vi "Instrument Manager Loop.vi"(8 "System Control":refnum<queue>, 11 "Instrument Manager":refnum<queue>) -> (0 "error out":errorcluster)   [LabVIEW 2020, in "Rename to match project.lvlib" / "Instrument Manager.lvlib"]
uses:
  Instrument Manager/Instrument Manager.lvlib
  support/Message Queue/Message Cluster.ctl
  Instrument Manager/Instrument State.ctl
  <vilib>/Utility/error.llb/Error Cluster From Error Code.vi
  <vilib>/ErrorRing/Error Ring.xnode
  support/Message Queue/Message Queue.lvlib
  Rename to match project.lvlib
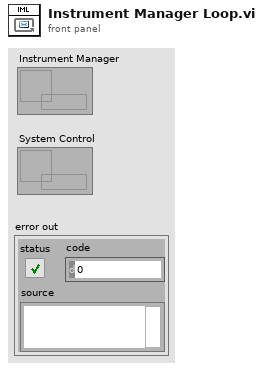
[diagram p1: front panel]
types:
  T1 = typedef "Rename to match project.lvlib/Instrument Manager.lvlib/Instrument State.ctl" = cluster{"VISA Resource":refnum<visa-resource-name>, "Setpoint":dbl, "Running":bool, "Running Since":timestamp, "Example Value Data Point":cluster{"Time Stamp":timestamp, "Value":dbl}, "Sampling Rate (sec/sample)":dbl}
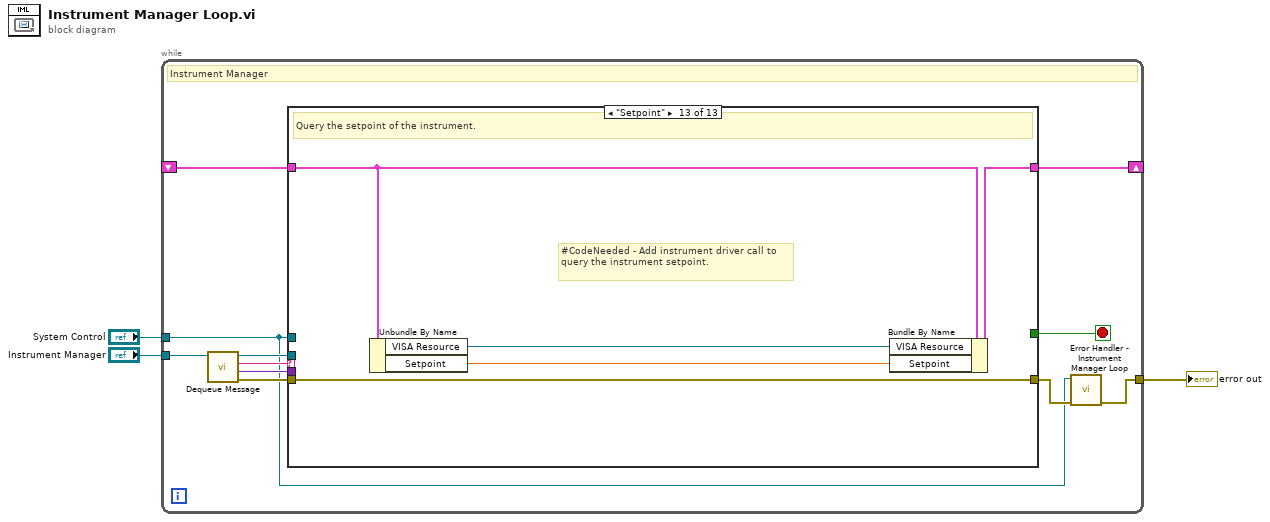
[diagram p0: block diagram]
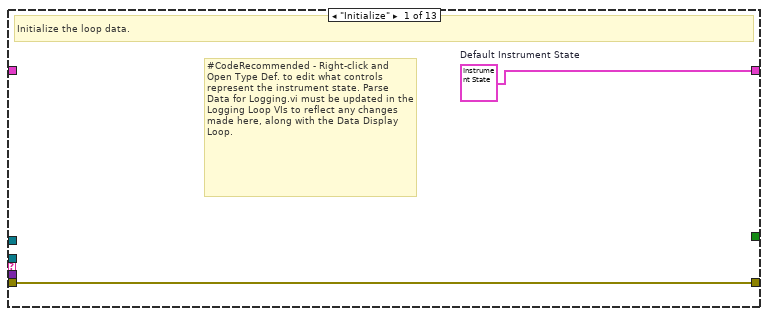
[diagram p2: hidden frame]
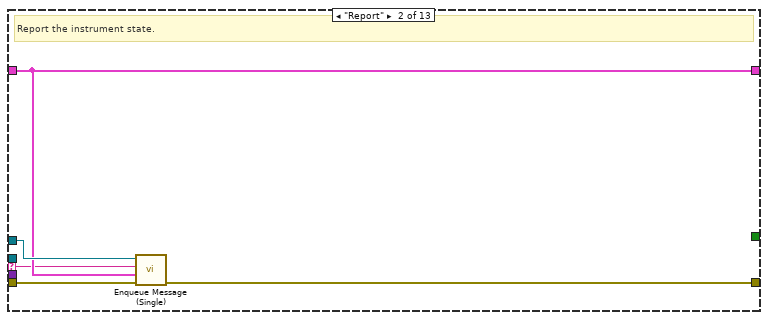
[diagram p3: hidden frame]
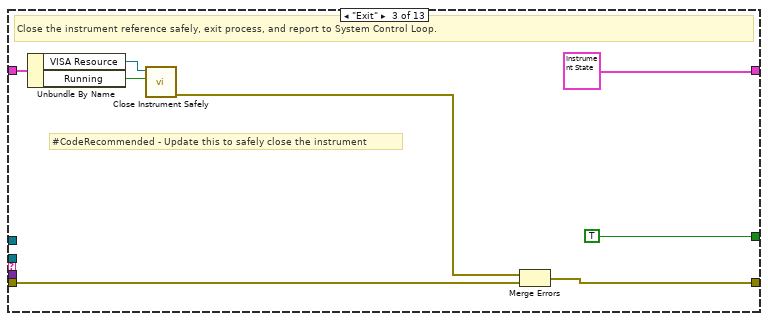
[diagram p4: hidden frame]
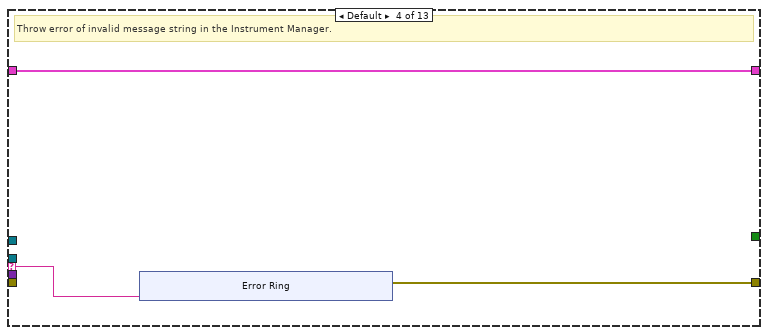
[diagram p5: hidden frame]
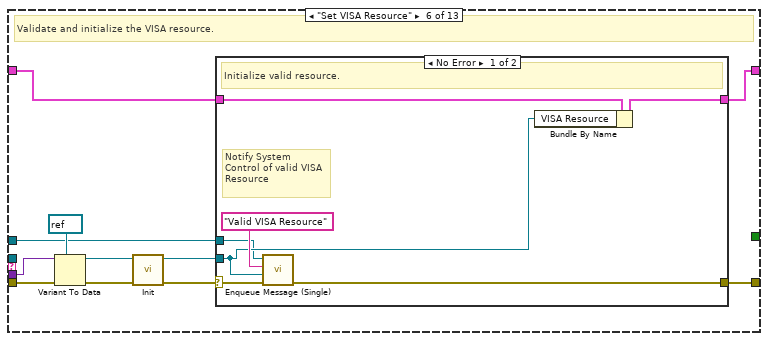
[diagram p7: hidden frame]
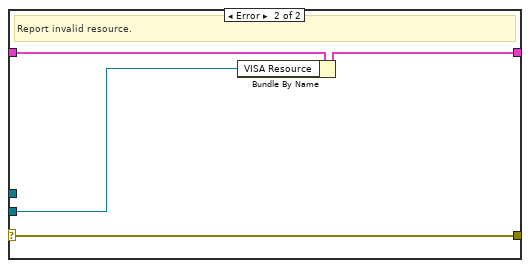
[diagram p8: hidden frame]
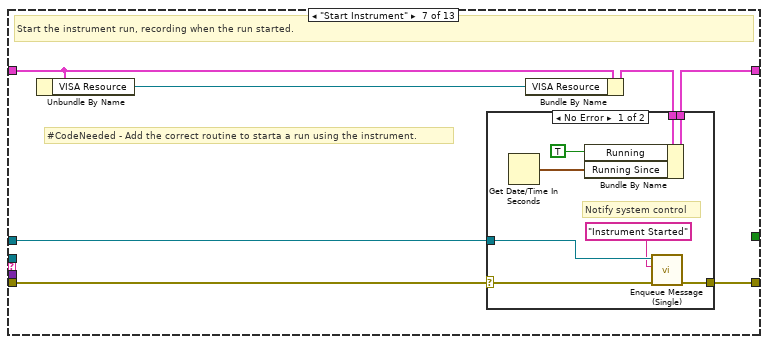
[diagram p9: hidden frame]
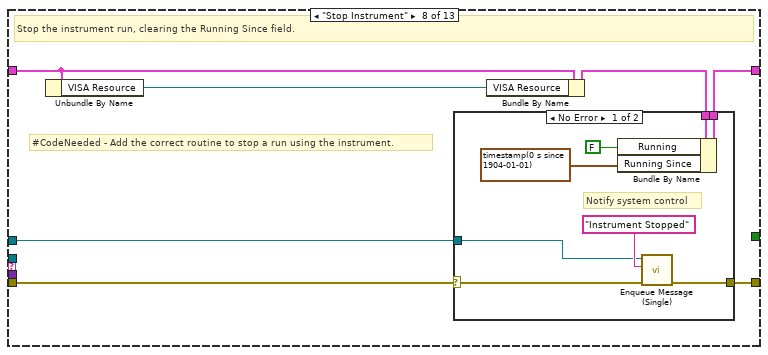
[diagram p11: hidden frame]
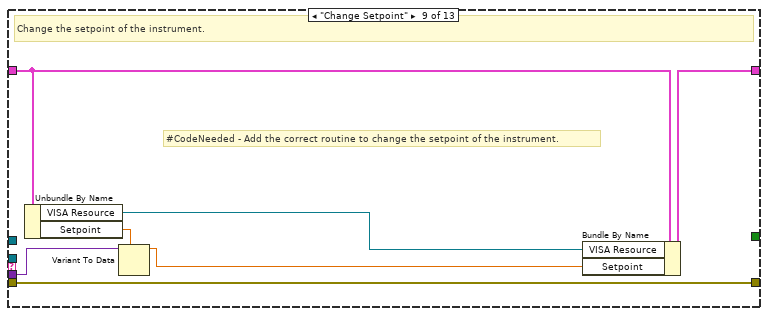
[diagram p13: hidden frame]
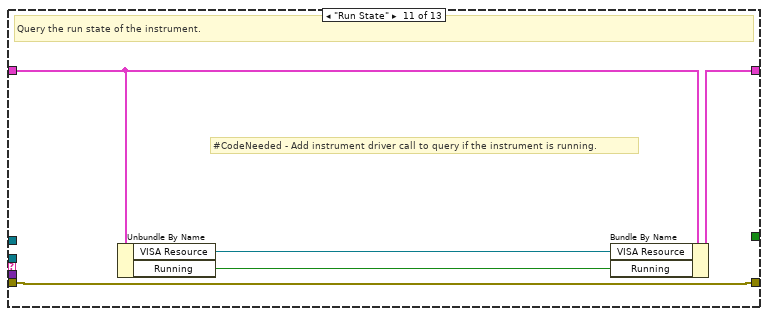
[diagram p15: hidden frame]
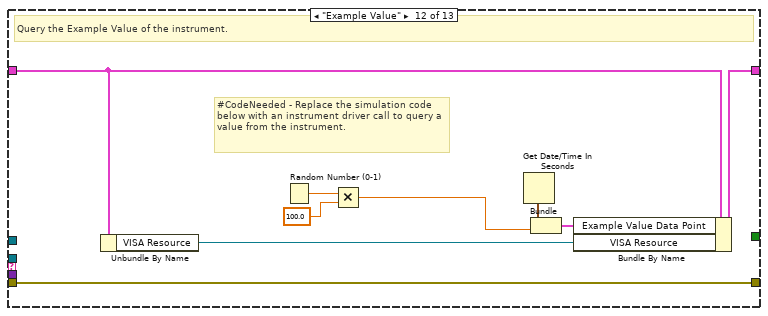
[diagram p16: hidden frame]
diagram:
  n1 = while {
    tunnel: "Instrument Manager" -> [w14]
    tunnel: "System Control" -> [w4]
    tunnel: [w8] -> w1
    shift-right: [w6] -> _
    shift-left: _ -> [w7]
    stop <- w5 stop-if-true
    # "Instrument Manager"
    n2 = call "Dequeue Message.vi"("Message Queue"=w14) -> ("error out"=w10:errorcluster, "Message Data"=w11:variant, "Message"=w13:string, "dup Message Queue"=w12:refnum<queue>)  [unwired: 7 in]
    n3 = case shown="\"Setpoint\"" w13 {
      selector: w13 -> [_ w17 _ w31 _ _ _ _ _ _ _ _ _]
      tunnel: w12 -> [_ _ _ _ _ _ _ _ _ _ _ _ _]
      tunnel: w4 -> [_ w20 _ _ _ w42 w69 w86 _ _ _ _ _]
      tunnel: w11 -> [_ _ _ _ _ w49 _ _ w103 _ _ _ _]
      tunnel: w10 -> [w16 w21 w24 _ w40 w48 w67 w84 w99 w106 w110 w116 w125]
      tunnel: [w16 w19 w23 w30 w40 w52 w70 w87 w99 w106 w110 w116 w125] -> w9
      tunnel: w7 -> [_ w18 w29 w32 w41 w51 w66 w83 w102 w105 w109 w117 w123]
      tunnel: [w15 w18 T1 {"VISA Resource"="", "Setpoint"=0.0, "Running"=FALSE, "Running Since"=timestamp(0 s since 1904-01-01), "Example Value Data Point"={"Time Stamp"=timestamp(0 s since 1904-01-01), "Value"=0.0}, "Sampling Rate (sec/sample)"=0.0} w32 w41 w50 w68 w85 w104 w105 w111 w120 w124] -> w6
      tunnel: [_ _ TRUE _ _ _ _ _ _ _ _ _ _] -> w5
      frame "Initialize" {
        w15 = T1 {"VISA Resource"="", "Setpoint"=0.0, "Running"=FALSE, "Running Since"=timestamp(0 s since 1904-01-01), "Example Value Data Point"={"Time Stamp"=timestamp(0 s since 1904-01-01), "Value"=0.0}, "Sampling Rate (sec/sample)"=0.0}  # Default Instrument State
        # "#CodeRecommended - Right-click and Open Type Def. to edit what controls represent the instrument state. Parse Data for Logging.vi must be updated in the Logging Loop VIs to reflect any changes made here, along with the Data Display Loop."
        # "Initialize the loop data."
      }
      frame "Report" {
        # "Report the instrument state."
        n4 = call "Enqueue Message (Single).vi"("error in (no error)"=w21, "Message Data"=w18, "Message"=w17, "Message Queue"=w20) -> ("error out"=w19:errorcluster)  [unwired: 6 in, 1 out]
      }
      frame "Exit" {
        # "#CodeRecommended - Update this to safely close the instrument"
        # "Close the instrument reference safely, exit process, and report to System Control Loop."
        n5 = Unbundle By Name(w29) -> ("VISA Resource"=w27:refnum<visa-resource-name>, "Running"=w28:bool)
        n6 = call "Close Instrument Safely.vi"("Running (F)"=w28, "VISA Refnum in"=w27) -> ("error out"=w22:errorcluster)  [unwired: 9 in]
        n7 = Merge Errors(w22, w24) -> (w23:errorcluster)
      }
      frame Default {
        # "Throw error of invalid message string in the Instrument Manager."
        n8 = xnode "Error Ring"("parameter 0"=w31) -> ("error out"=w30:errorcluster)
      }
      frame "--- Copy This Frame ---" {
        # "Copy this frame and add responses to instrument specific messages."
      }
      frame "Set VISA Resource" {
        # "Validate and initialize the VISA resource."
        n9 = Variant To Data(error in=w48, type=refnum<visa-resource-name> refnum, Variant=w49) -> (data=w46:refnum<visa-resource-name>, error out=w47:errorcluster)
        n10 = call "Init.vi"("error in (no error)"=w47, "VISA resource in"=w46) -> ("error out"=w43:errorcluster, "VISA resource out"=w44:refnum<visa-resource-name>)  [unwired: 8 in]
        n11 = case shown="No Error" w43 {
          selector: w43 -> [w59 w60]
          tunnel: w44 -> [w55 w61]
          tunnel: [w56 w60] -> w52
          tunnel: w51 -> [w53 w63]
          tunnel: [w57 w62] -> w50
          tunnel: w42 -> [w54 _]
          frame No Error {
            # "Notify System Control of valid VISA Resource"
            # "Initialize valid resource."
            n12 = call "Enqueue Message (Single).vi"("error in (no error)"=w59, "Message Data"=w55, "Message"="Valid VISA Resource", "Message Queue"=w54) -> ("error out"=w56:errorcluster)  [unwired: 6 in, 1 out]
            n13 = Bundle By Name(cluster=w53, "VISA Resource"=w55) -> (w57:T1)
          }
          frame Error {
            # "Report invalid resource."
            n14 = Bundle By Name(cluster=w63, "VISA Resource"=w61) -> (w62:T1)
          }
        }
      }
      frame "Start Instrument" {
        # "#CodeNeeded - Add the correct routine to starta a run using the instrument."
        # "Start the instrument run, recording when the run started."
        n15 = Unbundle By Name(w66) -> ("VISA Resource"=w64:refnum<visa-resource-name>)
        n16 = Bundle By Name(cluster=w66, "VISA Resource"=w64) -> (w65:T1)
        n17 = case shown="No Error" w67 {
          selector: w67 -> [w71 w80]
          tunnel: [w78 w80] -> w70
          tunnel: w69 -> [w77 _]
          tunnel: [w75 w79] -> w68
          tunnel: w65 -> [w72 w79]
          frame No Error {
            # "Notify system control"
            n18 = Get Date/Time In Seconds() -> (seconds since 1Jan1904=w73:timestamp)
            n19 = Bundle By Name(cluster=w72, "Running"=TRUE, "Running Since"=w73) -> (w75:T1)
            n20 = call "Enqueue Message (Single).vi"("error in (no error)"=w71, "Message"="Instrument Started", "Message Queue"=w77) -> ("error out"=w78:errorcluster)  [unwired: 7 in, 1 out]
          }
          frame Error {
          }
        }
      }
      frame "Stop Instrument" {
        # "#CodeNeeded - Add the correct routine to stop a run using the instrument."
        # "Stop the instrument run, clearing the Running Since field."
        n21 = Unbundle By Name(w83) -> ("VISA Resource"=w81:refnum<visa-resource-name>)
        n22 = Bundle By Name(cluster=w83, "VISA Resource"=w81) -> (w82:T1)
        n23 = case shown="No Error" w84 {
          selector: w84 -> [w88 w97]
          tunnel: w82 -> [w95 w96]
          tunnel: [w94 w97] -> w87
          tunnel: w86 -> [w92 _]
          tunnel: [w91 w96] -> w85
          frame No Error {
            # "Notify system control"
            n24 = Bundle By Name(cluster=w95, "Running"=FALSE, "Running Since"=timestamp(0 s since 1904-01-01)) -> (w91:T1)
            n25 = call "Enqueue Message (Single).vi"("error in (no error)"=w88, "Message"="Instrument Stopped", "Message Queue"=w92) -> ("error out"=w94:errorcluster)  [unwired: 7 in, 1 out]
          }
          frame Error {
          }
        }
      }
      frame "Change Setpoint" {
        # "#CodeNeeded - Add the correct routine to change the setpoint of the instrument."
        # "Change the setpoint of the instrument."
        n26 = Unbundle By Name(w102) -> ("VISA Resource"=w98:refnum<visa-resource-name>, "Setpoint"=w101:dbl)
        n27 = Variant To Data(type=w101, Variant=w103) -> (data=w100:dbl)  [unwired: 1 in, 1 out]
        n28 = Bundle By Name(cluster=w102, "VISA Resource"=w98, "Setpoint"=w100) -> (w104:T1)
      }
      frame "--- Copy for Get State Messages ---" {
        # "#CodeNeeded - Use the Bundle by Name function to bundle the new state value into the Instrument State cluster."
        # "#CodeNeeded - Add instrument driver call to query the instrument state requested"
        # "Duplicate this case for messages cases that will query the instrument state."
      }
      frame "Run State" {
        # "#CodeNeeded - Add instrument driver call to query if the instrument is running."
        # "Query the run state of the instrument."
        n29 = Unbundle By Name(w109) -> ("VISA Resource"=w108:refnum<visa-resource-name>, "Running"=w107:bool)
        n30 = Bundle By Name(cluster=w109, "VISA Resource"=w108, "Running"=w107) -> (w111:T1)
      }
      frame "Example Value" {
        # "#CodeNeeded - Replace the simulation code below with an instrument driver call to query a value from the instrument."
        # "Query the Example Value of the instrument."
        n31 = Unbundle By Name(w117) -> ("VISA Resource"=w115:refnum<visa-resource-name>)
        n32 = Random Number (0-1)() -> (number: 0 to 1=w114:dbl)
        n33 = Multiply(x=w114, y=100.0) -> (x*y=w112:dbl)
        n34 = Get Date/Time In Seconds() -> (seconds since 1Jan1904=w119:timestamp)
        n35 = Bundle("seconds since 1Jan1904"=w119, w112) -> (w118:cluster{"seconds since 1Jan1904":timestamp, dbl})  [unwired: 1 in]
        n36 = Bundle By Name(cluster=w117, "Example Value Data Point"=w118, "VISA Resource"=w115) -> (w120:T1)
      }
      frame "Setpoint" {
        # "#CodeNeeded - Add instrument driver call to query the instrument setpoint."
        # "Query the setpoint of the instrument."
        n37 = Unbundle By Name(w123) -> ("VISA Resource"=w122:refnum<visa-resource-name>, "Setpoint"=w121:dbl)
        n38 = Bundle By Name(cluster=w123, "VISA Resource"=w122, "Setpoint"=w121) -> (w124:T1)
      }
    }
    n39 = call "Error Handler - Instrument Manager Loop.vi"("error in (no error)"=w9, "Message Queue"=w4) -> ("dup error in"=w8:errorcluster)  [unwired: 8 in, 1 out]
  }
  "error out" <- w1
